vi "GetOphirHandle.vi"(2 "error in (no error)":errorcluster) -> (0 "error out":errorcluster, 1 "OphirRef Out":T1)   [LabVIEW 2012]
uses:
  TypeDefs/OphirRef.ctl
panel:
  in  "OphirCom":refnum<k7>
  out "headName":string
  out "headType":string
  out "serialNumber":string
  out "SerialNumber":string
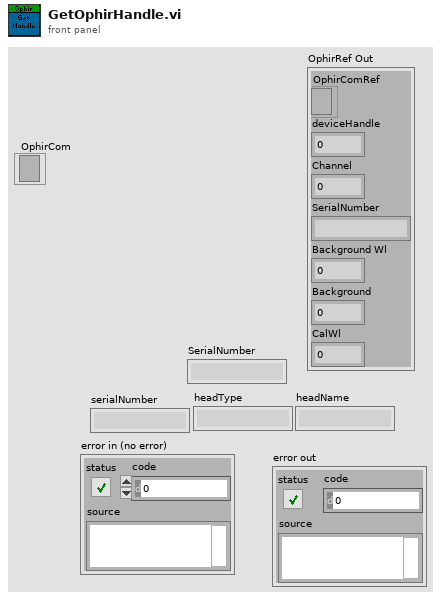
[diagram p1: front panel]
types:
  T1 = typedef "OphirRef.ctl" = cluster{"OphirComRef":refnum<k7>, "deviceHandle":i32, "Channel":i32, "SerialNumber":string, "Background Wl":dbl, "Background":dbl, "CalWl":dbl}
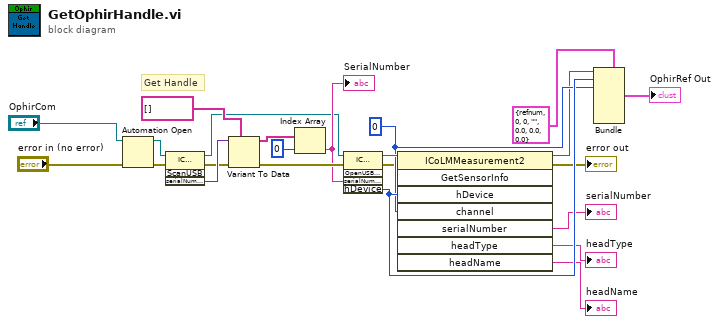
[diagram p0: block diagram]
diagram:
  w8 = 0 ("Channel")
  # "Get Handle"
  n1 = Automation Open(error in (no error)="error in (no error)", Automation Refnum="OphirCom") -> (Automation Refnum=w23:refnum<k7>, error out=w18:errorcluster)  [unwired: 2 in]
  n2 = invoke class="ICoLMMeasurement2" method="ScanUSB"(reference=w23, error in=w18) -> (reference out=w13:refnum<k7>, error out=w19:errorcluster, "serialNumbers"=w22:variant)  [unwired: 2 in, 1 out]
  n3 = Variant To Data(error in=w19, type=string[] [], Variant=w22) -> (data=w20:string[], error out=w16:errorcluster)
  n4 = Index Array(array=w20, index=0) -> (element=w15:string)
  "SerialNumber" <- w15
  n5 = invoke class="ICoLMMeasurement2" method="OpenUSBDevice"(reference=w13, error in=w16, "serialNumber"=w15) -> (reference out=w10:refnum<k7>, error out=w3:errorcluster, "hDevice"=w9:i32)  [unwired: 2 in, 2 out]
  n6 = invoke class="ICoLMMeasurement2" method="GetSensorInfo"(reference=w10, error in=w3, "hDevice"=w9, "channel"=w8) -> (reference out=w1:refnum<k7>, error out=→"error out":errorcluster, "serialNumber"=→"serialNumber":string, "headType"=→"headType":string, "headName"=→"headName":string)  [unwired: 4 in, 3 out]
  n7 = Bundle(cluster=T1 {"OphirComRef"=refnum, "deviceHandle"=0, "Channel"=0, "SerialNumber"="", "Background Wl"=0.0, "Background"=0.0, "CalWl"=0.0} ("output cluster"), "OphirComRef"=w1, "deviceHandle"=w9, "Channel"=w8) -> (→"OphirRef Out":T1)  [unwired: 4 in]
